vi "CalculateHighRateFeatures.vi"(7 "channels":T4[](array[typedef]), 8 "error in (no error)":errorcluster, 9 "pulse positions array":T3[](array[typedef]), 10 "waveforms":T2, 11 "Map":T1) -> (0 "error out":errorcluster, 5 "channels out":T4[](array[typedef]))   [LabVIEW 2017, in "AnalysisHelper.lvlib"]
uses:
  <vilib>/addons/InsightCM/Utilities/Analysis/Shared/AnalysisHelper.lvlib
  <vilib>/addons/InsightCM/Utilities/Analysis/Shared/controls/Channel.ctl
  <vilib>/addons/InsightCM/Utilities/Analysis/Shared/controls/SpeedType.ctl
  <vilib>/addons/InsightCM/Utilities/Analysis/Shared/controls/Feature.ctl
  <vilib>/addons/InsightCM/Utilities/Analysis/Shared/controls/AmplitudeScale.ctl
  <vilib>/addons/InsightCM/Utilities/Analysis/Shared/controls/PulsePositions.ctl
  <vilib>/addons/InsightCM/Utilities/DataAccessors/controls/wfmSGL_DVR.ctl
  <vilib>/addons/PointValueMap/controls/PointMap.ctl
  <vilib>/addons/InsightCM/Utilities/ChannelStatus/ChannelStatus.lvlib
  <vilib>/addons/PointValueMap/PointValueMap.lvlib
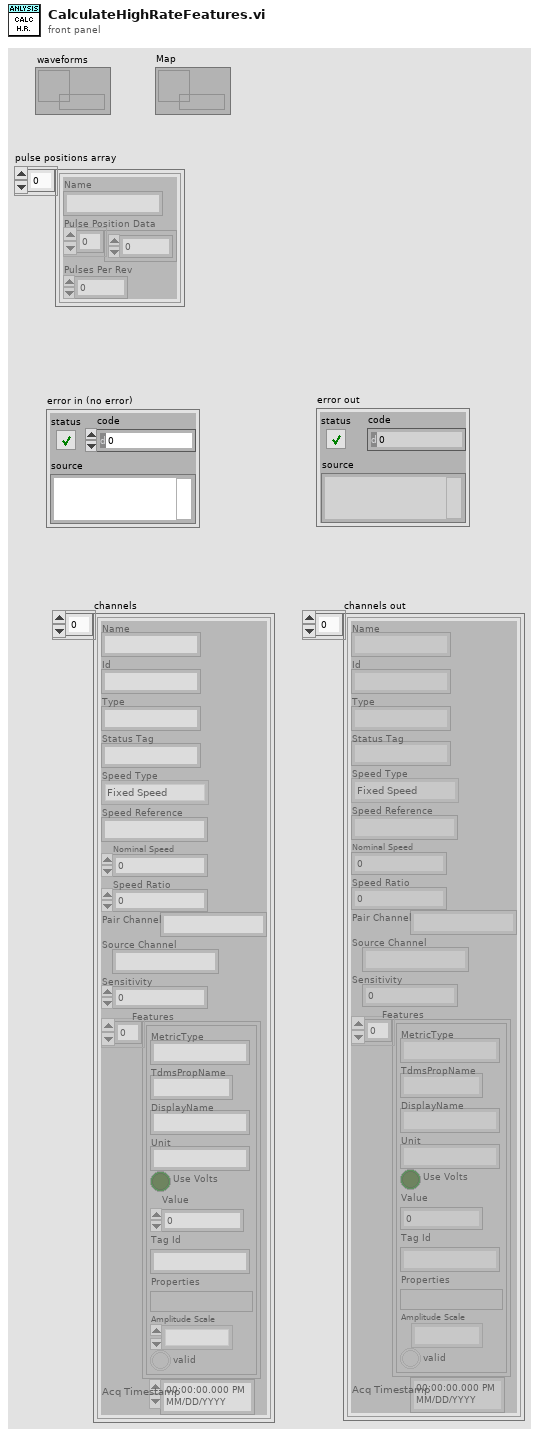
[diagram p1: front panel]
types:
  T1 = typedef "PointValueMap.lvlib/PointMap.ctl" = refnum<data-value>
  T2 = typedef "wfmSGL_DVR.ctl" = refnum<data-value>
  T3 = typedef "AnalysisHelper.lvlib/PulsePositions.ctl" = cluster{"Name":string, "Pulse Position Data":dbl[], "Pulses Per Rev":i32}
  T4 = typedef "AnalysisHelper.lvlib/Channel.ctl" = cluster{"Name":string, "Id":string, "Type":string, "Status Tag":string, "Speed Type":T5, "Speed Reference":string, "Nominal Speed":dbl, "Speed Ratio":dbl, "Pair Channel":string, "Source Channel":string, "Sensitivity":dbl, "Features":T6[], "Acq Timestamp":timestamp}
  T5 = typedef "AnalysisHelper.lvlib/SpeedType.ctl" = enum16{"Fixed Speed", "Tachometer", "From Map"}
  T6 = typedef "AnalysisHelper.lvlib/Feature.ctl" = cluster{"MetricType":string, "TdmsPropName":string, "DisplayName":string, "Unit":string, "Use Volts":bool, "Value":dbl, "Tag Id":string, "Properties":variant, "Amplitude Scale":T7, "valid":bool}
  T7 = typedef "AnalysisHelper.lvlib/AmplitudeScale.ctl" = enum16{"rms", "peak", "pk-pk"}
  T8 = typedef "AnalysisHelper.lvlib/LevelFeatures.ctl" = cluster{"RMS":dbl, "Peak":dbl, "Pk-Pk":dbl, "Derived Peak":dbl, "Crest Factor":dbl}
  T9 = typedef "AnalysisHelper.lvlib/MaxMinAvgFeatures.ctl" = cluster{"Max":dbl, "Min":dbl, "Avg":dbl}
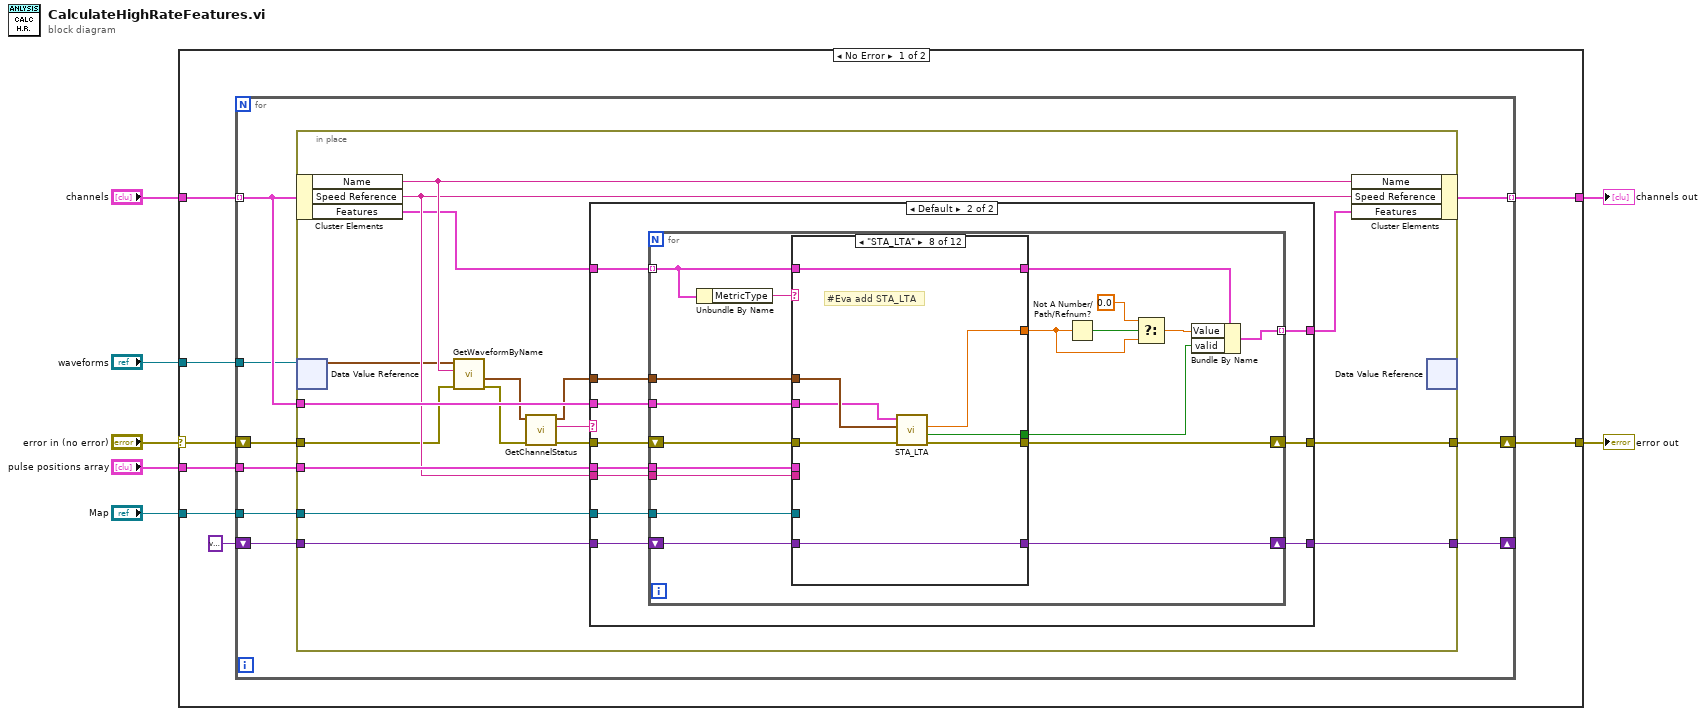
[diagram p0: block diagram]
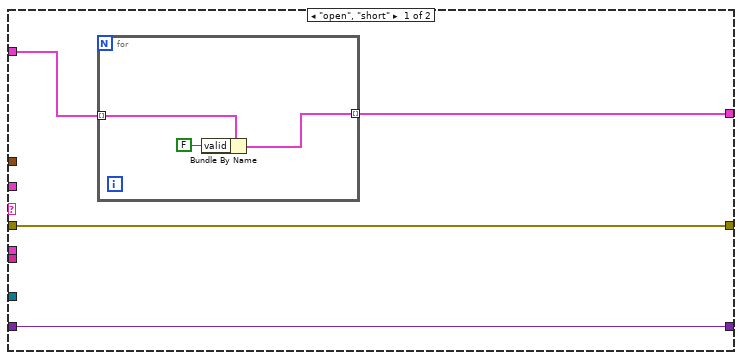
[diagram p2: hidden frame]
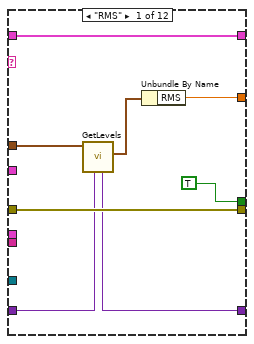
[diagram p3: hidden frame]
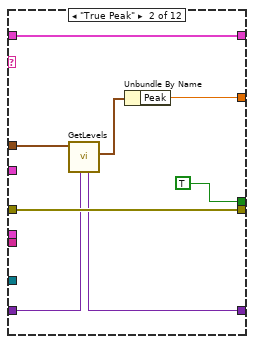
[diagram p4: hidden frame]
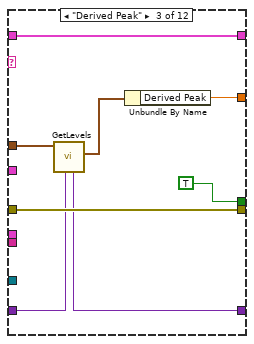
[diagram p5: hidden frame]
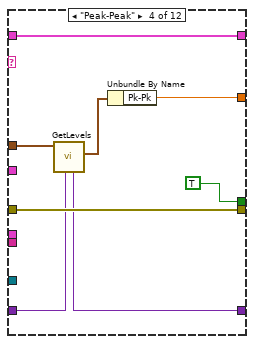
[diagram p6: hidden frame]
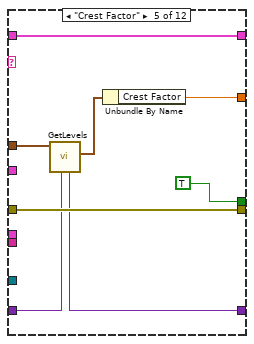
[diagram p7: hidden frame]
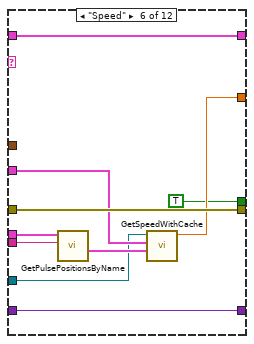
[diagram p8: hidden frame]
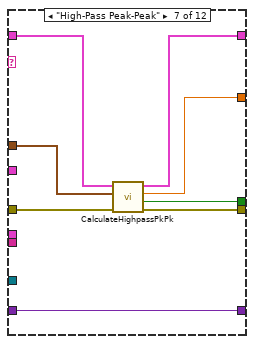
[diagram p9: hidden frame]
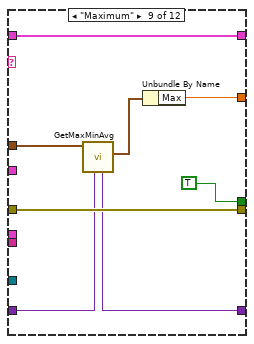
[diagram p10: hidden frame]
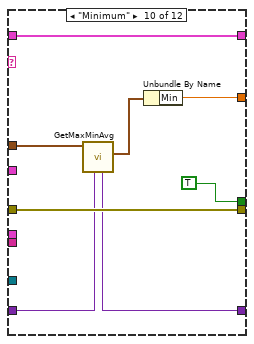
[diagram p11: hidden frame]
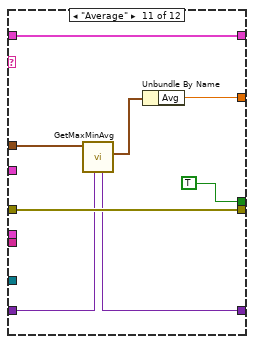
[diagram p12: hidden frame]
diagram:
  n1 = case shown="No Error" "error in (no error)" {
    selector: "error in (no error)" -> [w15 w171]
    tunnel: [w10 w171] -> w7
    tunnel: "channels" -> [w13 w172]
    tunnel: [w14 w172] -> w6
    tunnel: "pulse positions array" -> [w12 _]
    tunnel: "waveforms" -> [w9 _]
    tunnel: "Map" -> [w8 _]
    frame No Error {
      n2 = for {
        tunnel: w13 -> [w21] mode=indexing
        tunnel: [w24] -> w14 mode=indexing
        tunnel: w12 -> [w20]
        shift-right: [w18] -> _
        shift-left: variant -> [w19]
        shift-right: [w22] -> w10
        shift-left: w15 -> [w23]
        tunnel: w9 -> [w17]
        tunnel: w8 -> [w16]
        n3 = in-place {
          in-place-border: w23 -> [w34]
          in-place-border: [w41] -> w22
          in-place-border: w21 -> [w39]
          in-place-border: w20 -> [w36]
          in-place-border: w19 -> [w38]
          in-place-border: [w37] -> w18
          in-place-border: w16 -> [w25]
          n4 = in-place-cluster #1(w21) -> ("Name"=w40:string, "Speed Reference"=w35:string, "Features"=w33:T6[])
          n5 = in-place-dvr #2(w17) -> (w26:waveform(sgl)[])  [unwired: 1 out]
          n6 = call <vilib>:"GetWaveformByName.vi"("error in (no error)"=w34, "Channel Name"=w40, "Acq Waveforms"=w26) -> ("error out"=w31:errorcluster, "Waveform"=w28:waveform(sgl))  [unwired: 5 in, 2 out]
          n7 = call <vilib>:"GetChannelStatus.vi"("error in (no error)"=w31, "waveform in"=w28) -> ("error out"=w30:errorcluster, "channel status"=w29:string, "waveform out"=w27:waveform(sgl))  [unwired: 6 in, 1 out]
          n8 = case shown="Default" w29 {
            tunnel: [w42 w59] -> w32
            tunnel: w30 -> [w45 w58]
            tunnel: w33 -> [w43 w57]
            tunnel: w39 -> [_ w52]
            tunnel: w27 -> [_ w56]
            tunnel: [w45 w53] -> w41
            tunnel: w38 -> [w44 w55]
            tunnel: [w44 w54] -> w37
            tunnel: w36 -> [_ w51]
            tunnel: w35 -> [_ w50]
            tunnel: w25 -> [_ w49]
            frame "open", "short" {
              n9 = for {
                tunnel: w43 -> [w48] mode=indexing
                tunnel: [w46] -> w42 mode=indexing
                n10 = Bundle By Name(cluster=w48, "valid"=FALSE) -> (w46:T6)
              }
            }
            frame Default {
              n11 = for {
                tunnel: w57 -> [w72] mode=indexing
                tunnel: w56 -> [w76]
                tunnel: [w77] -> w59 mode=indexing
                tunnel: w52 -> [w73]
                shift-right: [w69] -> w54
                shift-left: w55 -> [w70]
                shift-right: [w74] -> w53
                shift-left: w58 -> [w75]
                tunnel: w51 -> [w68]
                tunnel: w50 -> [w67]
                tunnel: w49 -> [w60]
                n12 = Unbundle By Name(w72) -> ("MetricType"=w71:string)
                n13 = case shown="\"STA_LTA\"" w71 {
                  tunnel: [w82 w90 w98 w106 w114 w123 w131 w139 w150 w158 w166 _] -> w64
                  tunnel: w76 -> [w84 w91 w99 w107 w115 _ w134 w141 w147 w155 w163 _]
                  tunnel: w75 -> [w85 w93 w101 w109 w117 w127 w133 w140 w151 w159 w167 w169]
                  tunnel: [w85 w93 w101 w109 w117 w127 w132 w137 w151 w159 w167 w169] -> w74
                  tunnel: w73 -> [_ _ _ _ _ w124 _ w136 _ _ _ _]
                  tunnel: w72 -> [w79 w87 w95 w103 w111 w120 w130 w142 w149 w157 w165 w168]
                  tunnel: w70 -> [w81 w89 w97 w105 w113 w126 w135 w143 w146 w154 w162 w170]
                  tunnel: [w80 w88 w96 w104 w112 w126 w135 w143 w145 w153 w161 w170] -> w69
                  tunnel: w68 -> [_ _ _ _ _ w122 _ _ _ _ _ _]
                  tunnel: w67 -> [_ _ _ _ _ w121 _ _ _ _ _ _]
                  tunnel: [w79 w87 w95 w103 w111 w120 w129 w142 w149 w157 w165 w168] -> w62
                  tunnel: [TRUE ("valid") TRUE ("valid") TRUE ("valid") TRUE ("valid") TRUE ("valid") TRUE ("valid") w128 w138 TRUE ("valid") TRUE ("valid") TRUE ("valid") _] -> w61
                  tunnel: w60 -> [_ _ _ _ _ w118 _ _ _ _ _ _]
                  frame "RMS" {
                    n14 = call <vilib>:"GetLevels.vi"("calc cache"=w81, "waveform"=w84) -> ("levels"=w83:T8, "calc cache out"=w80:variant)  [unwired: 8 in]
                    n15 = Unbundle By Name(w83) -> ("RMS"=w82:dbl)
                  }
                  frame "True Peak" {
                    n16 = call <vilib>:"GetLevels.vi"("calc cache"=w89, "waveform"=w91) -> ("levels"=w92:T8, "calc cache out"=w88:variant)  [unwired: 8 in]
                    n17 = Unbundle By Name(w92) -> ("Peak"=w90:dbl)
                  }
                  frame "Derived Peak" {
                    n18 = call <vilib>:"GetLevels.vi"("calc cache"=w97, "waveform"=w99) -> ("levels"=w100:T8, "calc cache out"=w96:variant)  [unwired: 8 in]
                    n19 = Unbundle By Name(w100) -> ("Derived Peak"=w98:dbl)
                  }
                  frame "Peak-Peak" {
                    n20 = call <vilib>:"GetLevels.vi"("calc cache"=w105, "waveform"=w107) -> ("levels"=w108:T8, "calc cache out"=w104:variant)  [unwired: 8 in]
                    n21 = Unbundle By Name(w108) -> ("Pk-Pk"=w106:dbl)
                  }
                  frame "Crest Factor" {
                    n22 = call <vilib>:"GetLevels.vi"("calc cache"=w113, "waveform"=w115) -> ("levels"=w116:T8, "calc cache out"=w112:variant)  [unwired: 8 in]
                    n23 = Unbundle By Name(w116) -> ("Crest Factor"=w114:dbl)
                  }
                  frame "Speed" {
                    n24 = call <vilib>:"GetPulsePositionsByName.vi"("Channel Name"=w121, "Pulse Positions Array"=w122) -> ("Pulse Positions"=w125:T3)  [unwired: 6 in, 3 out]
                    n25 = call <vilib>:"GetSpeedWithCache.vi"("pulse positions"=w125, "channel"=w124, "Map"=w118) -> ("speed (RPM)"=w123:dbl)  [unwired: 7 in, 1 out]
                  }
                  frame "High-Pass Peak-Peak" {
                    n26 = call <vilib>:"CalculateHighpassPkPk.vi"("error in (no error)"=w133, "waveform in"=w134, "Feature"=w130) -> ("error out"=w132:errorcluster, "valid"=w128:bool, "value"=w131:dbl, "Feature out"=w129:T6)  [unwired: 5 in]
                  }
                  frame "STA_LTA" {
                    # "#Eva add STA_LTA"
                    n27 = call <vilib>:"STA_LTA.vi"("error in (no error)"=w140, "waveform in"=w141, "Channel Config"=w136) -> ("error out"=w137:errorcluster, "valid"=w138:bool, "value"=w139:dbl)  [unwired: 6 in]
                  }
                  frame "Maximum" {
                    n28 = call <vilib>:"GetMaxMinAvg.vi"("calc cache"=w146, "waveform"=w147) -> ("MaxMinAvg"=w144:T9, "calc cache out"=w145:variant)  [unwired: 8 in]
                    n29 = Unbundle By Name(w144) -> ("Max"=w150:dbl)
                  }
                  frame "Minimum" {
                    n30 = call <vilib>:"GetMaxMinAvg.vi"("calc cache"=w154, "waveform"=w155) -> ("MaxMinAvg"=w152:T9, "calc cache out"=w153:variant)  [unwired: 8 in]
                    n31 = Unbundle By Name(w152) -> ("Min"=w158:dbl)
                  }
                  frame "Average" {
                    n32 = call <vilib>:"GetMaxMinAvg.vi"("calc cache"=w162, "waveform"=w163) -> ("MaxMinAvg"=w160:T9, "calc cache out"=w161:variant)  [unwired: 8 in]
                    n33 = Unbundle By Name(w160) -> ("Avg"=w166:dbl)
                  }
                  frame Default {
                  }
                }
                n34 = Not A Number/Path/Refnum?(number/path/refnum=w64) -> (NaN/Path/Refnum?=w63:bool)
                n35 = Select(t=0.0, s=w63, f=w64) -> (s? t:f=w65:dbl)
                n36 = Bundle By Name(cluster=w62, "Value"=w65, "valid"=w61) -> (w77:T6)
              }
            }
          }
          n37 = in-place-cluster #1("Name"=w40, "Speed Reference"=w35, "Features"=w32) -> (w24:T4)
          n38 = in-place-dvr #2() -> ()  [unwired: 1 in, 2 out]
        }
      }
    }
    frame Error {
    }
  }
  "error out" <- w7
  "channels out" <- w6
